vi "Get Master Info.vi"(8 "error in (no error)":errorcluster, 11 "Item Ref in":T1 format="%.0x") -> (0 "error out":errorcluster, 1 "Master #":u32, 2 "Master Name":string, 3 "Item Ref out":T1 format="%.0x")   [LabVIEW 2019, in "SEECD System Explorer.lvlib"]
uses:
  SEECD System Explorer.lvlib
  <vilib>/NI VeriStand/Custom Device API/Custom Device Item Ref.ctl
  Shared/Globals/Property Strings.vi
  <vilib>/NI VeriStand/Custom Device API/Get Item Property (U32).vi
  <vilib>/NI VeriStand/Custom Device API/Custom Device API.lvlib
  Shared/SEECD Shared.lvlib
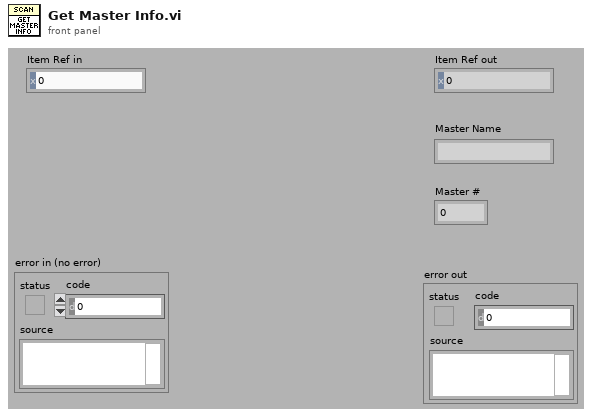
[diagram p1: front panel]
types:
  T1 = typedef "Custom Device API.lvlib/Custom Device Item Ref.ctl" = u64
  T2 = typedef "Custom Device API.lvlib/Custom Device Item Info.ctl" = cluster{"Name":string, "Is Channel":bool, "GUID":string, "Is Waveform":bool}
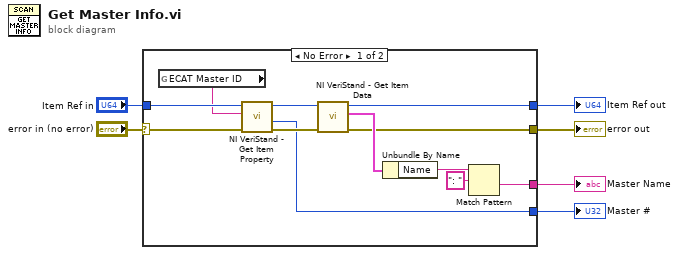
[diagram p0: block diagram]
diagram:
  n1 = case shown="No Error" "error in (no error)" {
    selector: "error in (no error)" -> [w17 w20]
    tunnel: [w10 w20] -> w5
    tunnel: "Item Ref in" -> [w18 w19]
    tunnel: [w11 w19] -> w3
    tunnel: [w9 _] -> w2
    tunnel: [w8 _] -> w1
    frame No Error {
      n2 = global read "Property Strings.vi" "ECAT Master ID"() -> (w7:string)
      n3 = call-poly <vilib>:"NI VeriStand - Get Item Property.vi"("error in (no error)"=w17, "Property Name"=w7, "Item Ref in"=w18) -> ("error out"=w12:errorcluster, "Value"=w8:u32, "Item Ref out"=w13:T1)  [unwired: 5 in, 1 out]
      n4 = call <vilib>:"NI VeriStand - Get Item Data.vi"("error in (no error)"=w12, "Item Ref in"=w13) -> ("error out"=w10:errorcluster, "Item Info"=w14:T2, "Item Ref out"=w11:T1)  [unwired: 7 out]
      n5 = Unbundle By Name(w14) -> ("Name"=w15:string)
      n6 = Match Pattern(string=w15, regular expression=": " ("search string/char (-)")) -> (after substring=w9:string)  [unwired: 1 in, 3 out]
    }
    frame Error {
    }
  }
  "error out" <- w5
  "Item Ref out" <- w3
  "Master #" <- w1
  "Master Name" <- w2
